vi "Stop Easing Prematurely.vi"(7 "Set or Get Value":enum16{"Set", "Get"}(ring), 11 "Stop?":bool) -> (3 "Stop?":bool)   [LabVIEW 2011, in "Sliding Menu Library.lvlib" / "Sliding Menu XControl.xctl"]
uses:
  Sliding Menu xControl/Sliding Menu XControl.xctl
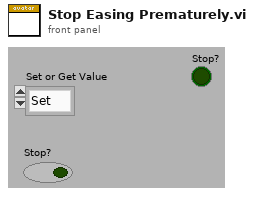
[diagram p1: front panel]
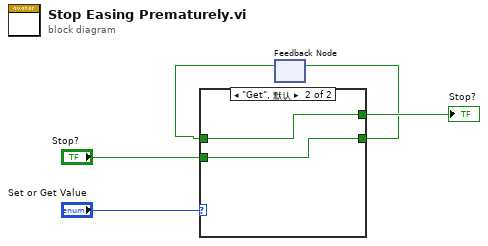
[diagram p0: block diagram]
diagram:
  n1 = feedback #1() -> (w1:bool)  [unwired: 1 in]
  n2 = case shown="\"Get\", 默认" "Set or Get Value" {
    tunnel: "Stop?" -> [w6 w7]
    tunnel: [w6 w7] -> w2
    tunnel: w1 -> [_ w8]
    tunnel: [w6 w8] -> w3
    frame "Set" {
    }
    frame "Get", Default {
    }
  }
  "Stop?" <- w3
  n3 = feedback-in #1(w2) -> ()
